vi "append_to_log.vi"(5 "data_type":T1, 7 "dims":T2, 8 "error in (no error)":errorcluster, 9 "Location":string, 10 "Data":variant, 11 "pcfs_hdf5_log in":refnum<class "pcfs_hdf5_log.lvclass">) -> (0 "error out":errorcluster, 3 "pcfs_hdf5_log out":refnum<class "pcfs_hdf5_log.lvclass">)   [LabVIEW 2015, in "pcfs_hdf5_log.lvclass"]
uses:
  pcfs_hdf5_log.lvclass
  Data Logger Class/data_dimensionality.ctl
  Data Logger Class/logger_data_types.ctl
  Detector_Class/Picoquant/Picoquant_generic/picoquant_data_tdef.ctl
  pcfs_hdf5_log.lvclass/pcfs_hdf5_log.ctl
  <vilib>/UPVI/lvhdf5/dataset.llb/Append Element(s) to Dataset (Variant).vi
  <vilib>/UPVI/lvhdf5/dataset.llb/Append Element(s) to Dataset.xnode
  <vilib>/UPVI/lvhdf5/library.llb/HDF5 Ref.ctl
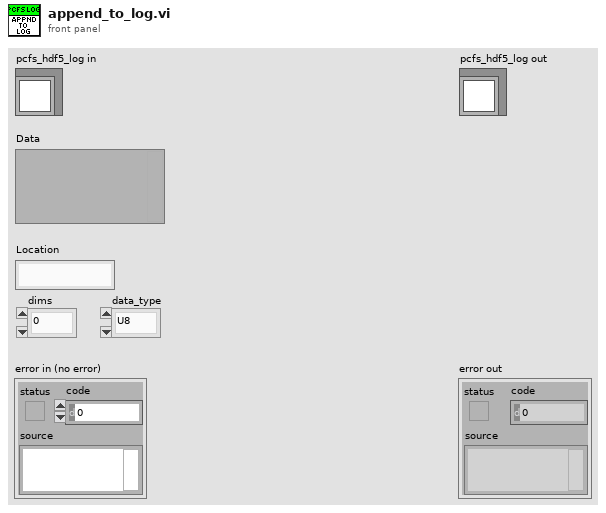
[diagram p1: front panel]
types:
  T1 = typedef "logger_data_types.ctl" = enum16{"U8", "I8", "U16", "I16", "U32", "I32", "DBL", "String"}
  T2 = typedef "data_dimensionality.ctl" = enum16{"0", "1", "2"}
  T3 = typedef "picoquant_data_tdef.ctl" = cluster{"channels":u8[], "times":u64[], "sync":u64[]}
  T4 = typedef "HDF5 Ref.ctl" = refnum<k1>
  T5 = typedef "hpanel_acq_modes.ctl" = u16
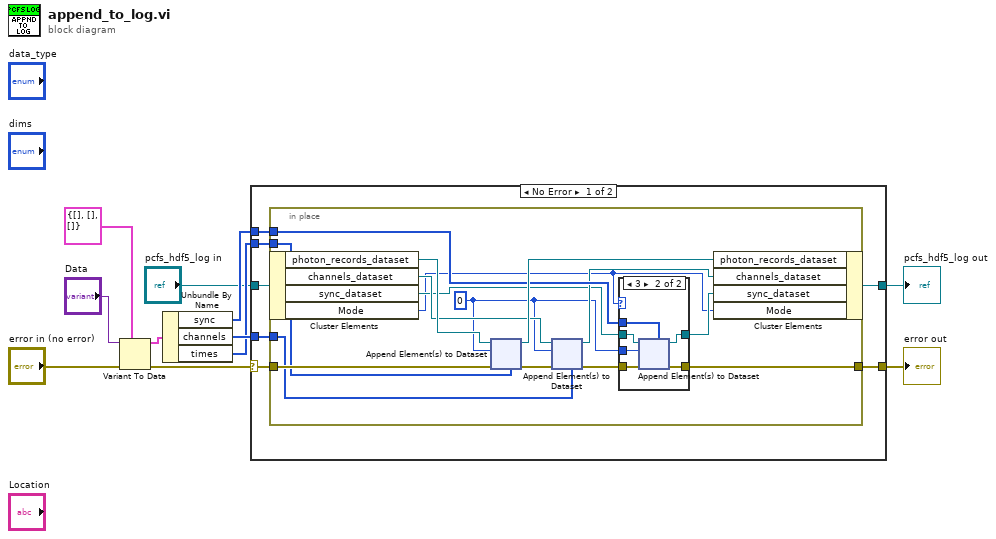
[diagram p0: block diagram]
diagram:
  n1 = Variant To Data(error in="error in (no error)", type=T3 {"channels"=[], "times"=[], "sync"=[]} ("data 2"), Variant="Data") -> (data=w9:T3, error out=w11:errorcluster)
  n2 = Unbundle By Name(w9) -> ("sync"=w8:u64[], "channels"=w7:u8[], "times"=w6:u64[])
  n3 = case shown="No Error" w11 {
    selector: w11 -> [w16 w67]
    tunnel: "pcfs_hdf5_log in" -> [w18 w66]
    tunnel: w7 -> [w17 _]
    tunnel: [w15 w67] -> w2
    tunnel: w6 -> [w14 _]
    tunnel: w8 -> [w13 _]
    tunnel: [w12 w66] -> w1
    frame No Error {
      n4 = in-place {
        in-place-border: w17 -> [w19]
        in-place-border: w16 -> [w29]
        in-place-border: [w28] -> w15
        in-place-border: w14 -> [w20]
        in-place-border: w13 -> [w27]
        w22 = 0 ("Dimension to Extend (0)")
        n5 = in-place-cluster #1(w18) -> ("photon_records_dataset"=w33:T4, "channels_dataset"=w26:T4, "sync_dataset"=w24:T4, "Mode"=w21:T5)
        n6 = xnode "Append Element(s) to Dataset"("Dimension to Extend (0)"=w22, "HDF5 Dataset Ref"=w33, "error in (no error)"=w29, "Data Element(s)"=w20) -> ("HDF5 Dataset out"=w32:T4, "error out"=w31:errorcluster)  [unwired: 2 out]
        n7 = xnode "Append Element(s) to Dataset"("Dimension to Extend (0)"=w22, "HDF5 Dataset Ref"=w26, "error in (no error)"=w31, "Data Element(s)"=w19) -> ("HDF5 Dataset out"=w25:T4, "error out"=w30:errorcluster)  [unwired: 2 out]
        n8 = case shown="3" w21 {
          tunnel: w30 -> [w35 w41]
          tunnel: [w35 w40] -> w28
          tunnel: w27 -> [_ w39]
          tunnel: w24 -> [w34 w38]
          tunnel: [w34 w37] -> w23
          tunnel: w22 -> [_ w36]
          frame 2, Default {
          }
          frame 3 {
            n9 = xnode "Append Element(s) to Dataset"("Dimension to Extend (0)"=w36, "HDF5 Dataset Ref"=w38, "error in (no error)"=w41, "Data Element(s)"=w39) -> ("HDF5 Dataset out"=w37:T4, "error out"=w40:errorcluster)  [unwired: 2 out]
          }
        }
        n10 = in-place-cluster #1("photon_records_dataset"=w32, "channels_dataset"=w25, "sync_dataset"=w23, "Mode"=w21) -> (w12:refnum<class "pcfs_hdf5_log.lvclass">)
      }
    }
    frame Error {
    }
  }
  "error out" <- w2
  "pcfs_hdf5_log out" <- w1
